vi "NRPM Measurement Error Codes.vi"(8 "error in (no error)":errorcluster, 9 "Sensor (1)":i32=1, 10 "Instance (1)":i32=1, 11 "VISA resource name":refnum<visa-resource-name>) -> (0 "error out":errorcluster, 1 "Error Code":i32[](array[numeric]), 2 "Reliability":i32, 3 "VISA resource name out":refnum<visa-resource-name>)   [LabVIEW 2015, in "Rohde&Schwarz CMXP GPRF.lvlib"]
doc: "Returns the measurement results for the power sensor connected to Sensor <no>.\n\nAttribute:\nRSCMXPGPRF_ATTR_NRPM_MEASUREMENT_SENSOR_POWER\n\nRemote-control command:\nFETCh:GPRF:MEAS<i>:NRPM:SENSor<no>:POWer?"
uses:
  <instrlib>/Rohde&Schwarz CMXP GPRF/Rohde&Schwarz CMXP GPRF.lvlib
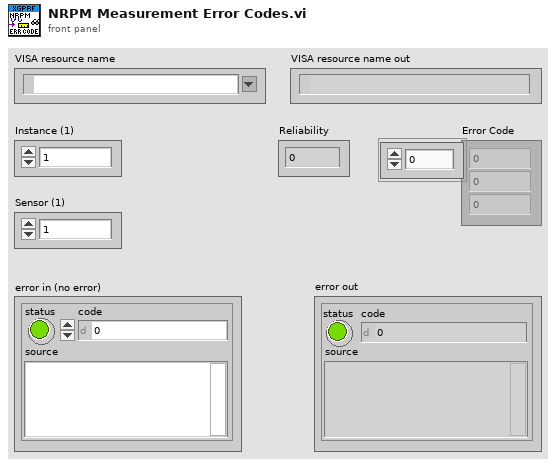
[diagram p1: front panel]
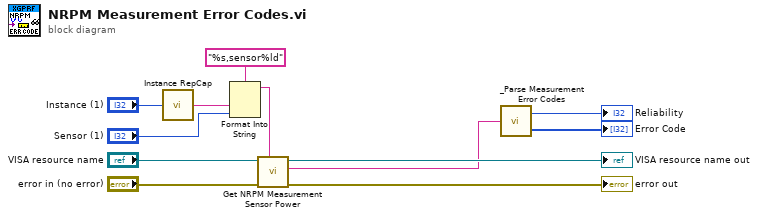
[diagram p0: block diagram]
diagram:
  n1 = call <instrlib>:"Instance RepCap.vi"("instance  in"="Instance (1)") -> ("instance out"=w10:string)
  n2 = Format Into String(format string="%s,sensor%ld", w10, "Sensor (1)") -> (resulting string=w7:string)  [unwired: 2 in, 1 out]
  n3 = call "Get NRPM Measurement Sensor Power"("Repeated Capabilities"=w7, "error in (no error)"="error in (no error)", "instrument handle"="VISA resource name") -> ("error out"=→"error out":errorcluster, "NRPM Measurement Sensor Power"=w1:string, "instrument handle out"=→"VISA resource name out":refnum<visa-resource-name>)  [unwired: 6 in]
  n4 = call <instrlib>:"_Parse Measurement Error Codes.vi"("String In"=w1) -> ("Reliability"=→"Reliability":i32, "Results"=→"Error Code":i32[])
